vi "FlagJSONTest.vi"(10 "State":bool[](array[boolean])) -> (0 "error out":errorcluster, 2 "Pass":bool)   [LabVIEW 2015]
uses:
  Flags/ColorEnum.ctl
  Flags/ColorFlags.ctl
  Flags/Flags.lvclass/Flags.ctl
  Flags/Read Color.vi
  Flags/Read State.vi
  Flags/Flags.lvclass
panel:
  out "RoomNumFlags":T1={"Flag State"=[1, 3, 5, 7]}
  in  "Color":T2[](array[typedef])=[enum."Red", enum."Blue", enum."Green", enum."Yellow"]
  out "After Json":bool[](array[boolean])
  out "Test Read":bool[](array[boolean])
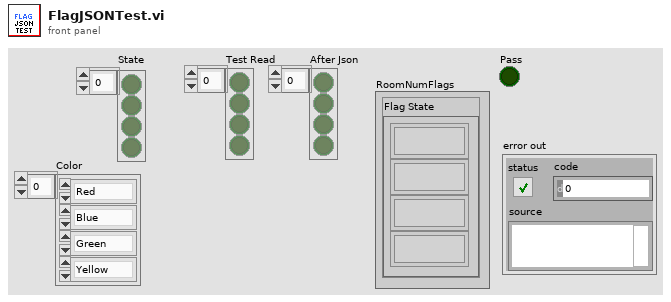
[diagram p1: front panel]
types:
  T1 = typedef "Flags.lvclass/ColorFlags.ctl" = cluster{"Flag State":u8[]}
  T2 = typedef "Flags.lvclass/ColorEnum.ctl" = enum8{"Red", "Blue", "Green", "Yellow"}
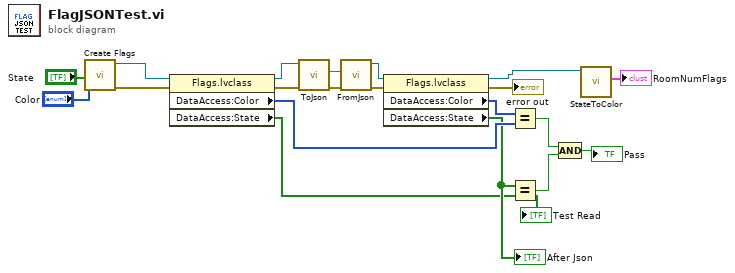
[diagram p0: block diagram]
diagram:
  n1 = call "Create Flags.vi"("Color"="Color", "State"="State") -> ("error out"=w3:errorcluster, "reference out"=w4:refnum<class "Flags.lvclass">)  [unwired: 8 in]
  n2 = property class="Flags.lvclass"(reference=w4, error in=w3) -> (reference out=w19:refnum<class "Flags.lvclass">, error out=w13:errorcluster, "DataAccess:Color"=w16:T2[], "DataAccess:State"=w8:bool[])
  "Test Read" <- w8
  n3 = call "ToJson.vi"("error in (no error)"=w13, "Flags in"=w19) -> ("error out"=w12:errorcluster, "String"=w20:string)  [unwired: 7 in, 1 out]
  n4 = call "FromJson.vi"("error in (no error)"=w12, "String"=w20) -> ("error out"=w11:errorcluster, "Flags out"=w18:refnum<class "Flags.lvclass">)  [unwired: 8 in]
  n5 = property class="Flags.lvclass"(reference=w18, error in=w11) -> (reference out=w2:refnum<class "Flags.lvclass">, error out=→"error out":errorcluster, "DataAccess:Color"=w17:T2[], "DataAccess:State"=w9:bool[])
  "After Json" <- w9
  n6 = Equal?(x=w17, y=w16) -> (x = y?=w15:bool)
  n7 = Equal?(x=w9, y=w8) -> (x = y?=w7:bool)
  n8 = Compound Arithmetic op=AND(w15, w7) -> (→"Pass":bool)
  n9 = call "StateToColor.vi"("Flags in"=w2) -> ("RoomNumFlags"=→"RoomNumFlags":T1)  [unwired: 8 in, 2 out]
